vi "DSC Alarm Event Example.vi"() -> ()   [LabVIEW 2018, in "Dynamic Shared Variables.lvlib"]
uses:
  Dynamic Shared Variables.lvlib
  Alarm Cluster (UI).ctl
  Alarm Cluster.ctl
  <vilib>/Utility/miscctls.llb/LVMouseTypeDef.ctl
  Tag VIs/Tag FGV Operation Enum.ctl
  Alarm Log Operation Enum.ctl
  <vilib>/lvdsc/NI_DSC.lvlib
  Waveform Loop/Waveform Loop.lvlib
panel:
  out "Alarm CSV Logfile path":path
  out "Alarm Event Time":timestamp
  in  "Tag Value":dbl=80.0 format="%#_13g"
  in  "Write Tag Value":bool
  in  "numeric alarm settings":T1={"enable? (F)"=TRUE, "name"="HiHi", "alarm type"=enum."HI_HI", "level/change"=50.0, "deadband/time"=1.0, "priority"=1, "ack type"=enum."Each Occurrence", "area"="", "description"="", "log? (T)"=TRUE}
  in  "Create Shared Variable":bool
  out "Alarm Model":T2[](array[typedef]) {"Alarm"."value" format="%.2f"; "Alarm"."setpoint" format="%.2f"; "Alarm"."clear time" format="%<%X\n%x>T"; "Alarm"."ack time" format="%<%X\n%x>T"; "Alarm"."set time" format="%<%X\n%x>T"}
  in  "Alarms":T3[](array[typedef])
  in  "stop":bool
  # "Instructions\n1. Press Create Shared Variable button with designated HI_HI threshold.\n2. Press Write Tag Value to write a Tag Value that is above the HI_HI threshold.\n3. Observe that the Alarm Event was triggered when the Alarm Event Time changes.\n4. Observer that the HIHi alarm is displayed in the alarm array."
  # "2."
  # "1."
  # "3."
  # "4."
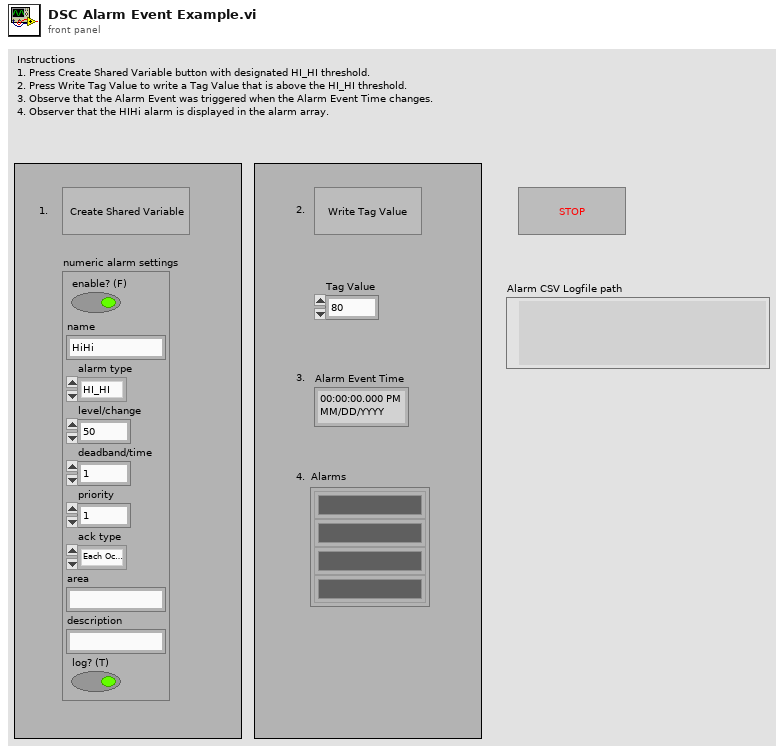
[diagram p1: front panel]
types:
  T1 = cluster{"enable? (F)":bool, "name":string, "alarm type":enum16{"HI_HI", "HI", "LO", "LO_LO"}, "level/change":dbl, "deadband/time":dbl, "priority":u32, "ack type":enum16{"Auto", "User", "None", "Each Occurrence"}, "area":string, "description":string, "log? (T)":bool}
  T2 = typedef "Dynamic Shared Variables.lvlib/Alarm Cluster.ctl" = cluster{"Color Box":u32, "Name":string, "Ack":bool, "Alarm":cluster{"alarm URL":string, "set time":timestamp, "set user":string, "ack time":timestamp, "ack user":string, "clear time":timestamp, "clear user":string, "setpoint":dbl, "value":dbl, "priority":u32, "alarm area":string, "alarm description":string, "ack comment":string, "event?":bool, "Refnum":u64}}
  T3 = typedef "Dynamic Shared Variables.lvlib/Alarm Cluster (UI).ctl" = cluster{"Color Box":u32, "Name":string, "Ack":bool}
  T4 = typedef "Alarm Log Operation Enum.ctl" = enum16{"Create Log", "Log Alarm", "Close Log"}
  T5 = typedef "Tag FGV Operation Enum.ctl" = enum16{"Init", "Set Notification Queue", "Create Tag", "Commit", "Write Tag (Numeric)", "Write Tag (Boolean)", "Read All Tags", "Read One Tag", "Delete Tag Category", "Set Alarm Parameters (Numeric)", "Set Alarm Parameters (Boolean)", "Enable All Alarms", "Disable All Alarms", "Delete All Tags", "Read Alarms", "Ack Alarm", "Read Alarm Parameters (Numeric)", "Read Alarm Parameters (Boolean)"}
  T6 = typedef "LVMouseTypeDef.ctl" = cluster{"Mouse Position":cluster{"X":i32, "Y":i32}, "Mouse Modifiers":cluster{"Button Down":bool, "Shift Mod":bool, "Menu Mod":bool, "Option Mod":bool}}
  T7 = cluster{"Down":bool, "Mouse":T6, "Drag":bool, "Canvas":bool}
  T8 = enum32{"u32BitField", "bool", "double", "string", "int8", "uint8", "int16", "uint16", "int32", "uint32", "int64", "uint64", "single", "double waveform", "int16 waveform", "array of boolean", "array of int8", "array of uint8", "array of int16", "array of uint16", "array of int32", "array of uint32", "array of int64", "array of uint64", "array of single", "array of double", "array of double waveform", "array of int16 waveform", "array of string", "variant", "timestamp", "fixed point", "custom"}
  T9 = cluster{"alarm URL":string, "set time":timestamp, "set user":string, "ack time":timestamp, "ack user":string, "clear time":timestamp, "clear user":string, "setpoint":dbl, "value":dbl, "priority":u32, "alarm area":string, "alarm description":string, "ack comment":string, "event?":bool, "Refnum":u64}[]
  T10 = cluster{"alarm URL":string, "set time":timestamp, "set user":string, "ack time":timestamp, "ack user":string, "clear time":timestamp, "clear user":string, "setpoint":dbl, "value":dbl, "priority":u32, "alarm area":string, "alarm description":string, "ack comment":string, "event?":bool, "Refnum":u64}
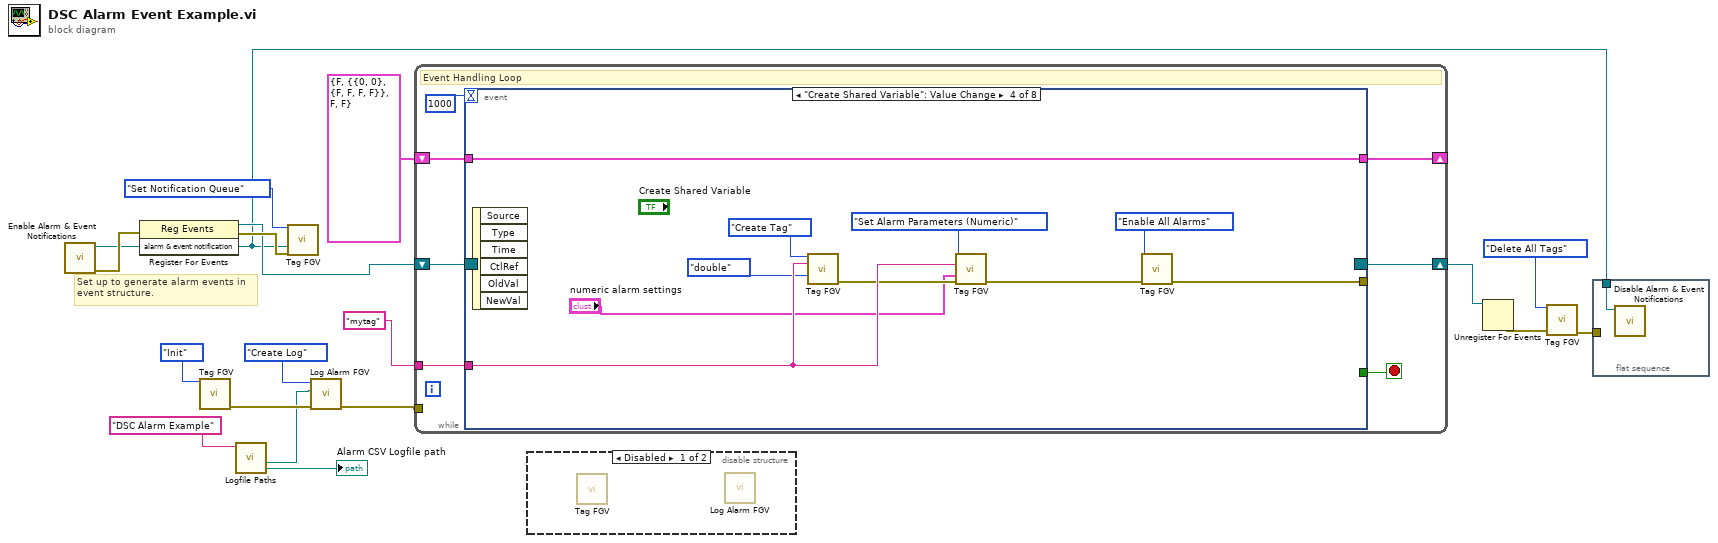
[diagram p0: block diagram]
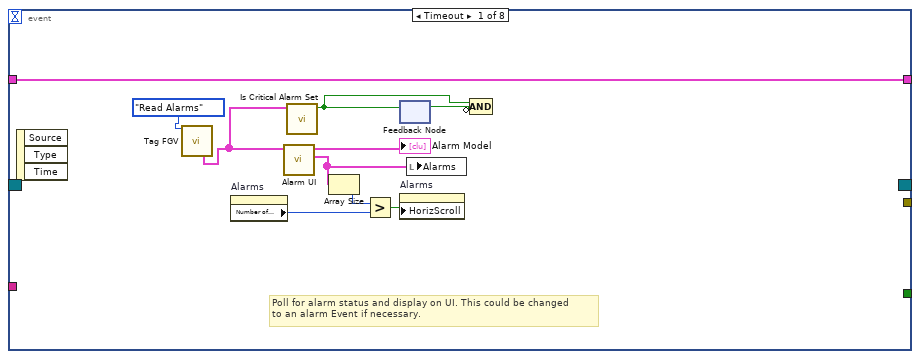
[diagram p3: hidden frame]
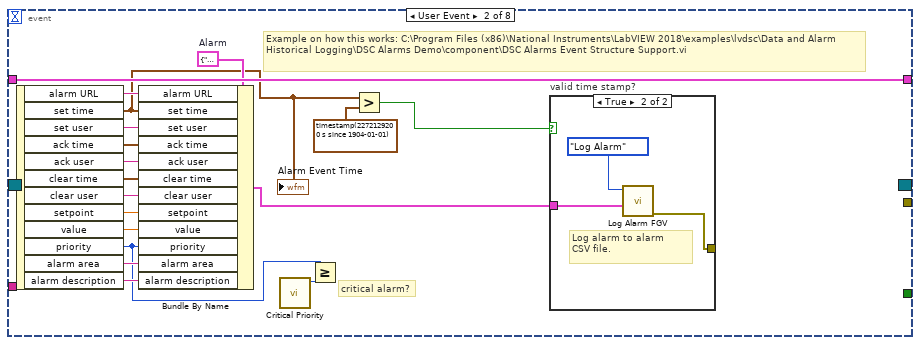
[diagram p4: hidden frame]
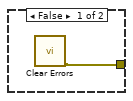
[diagram p5: hidden frame]
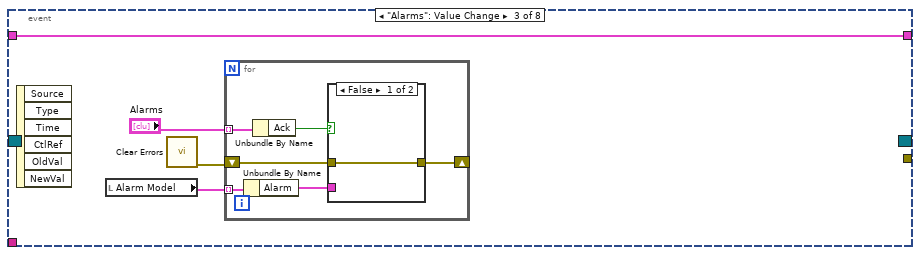
[diagram p6: hidden frame]
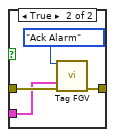
[diagram p7: hidden frame]
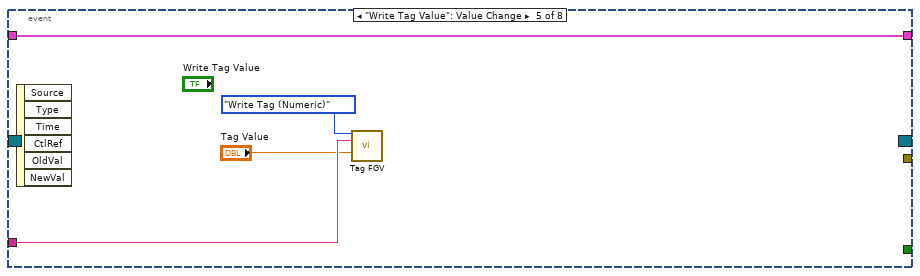
[diagram p8: hidden frame]
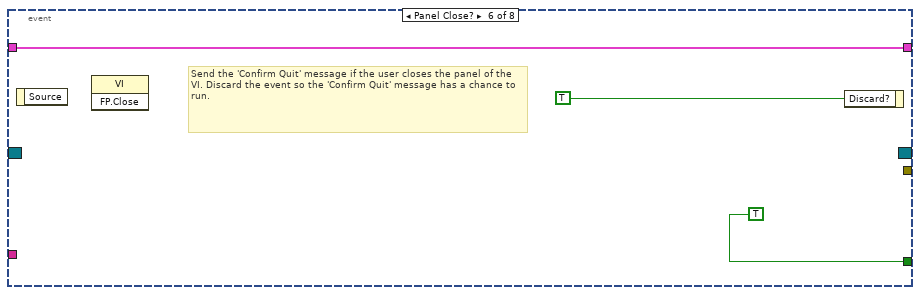
[diagram p9: hidden frame]
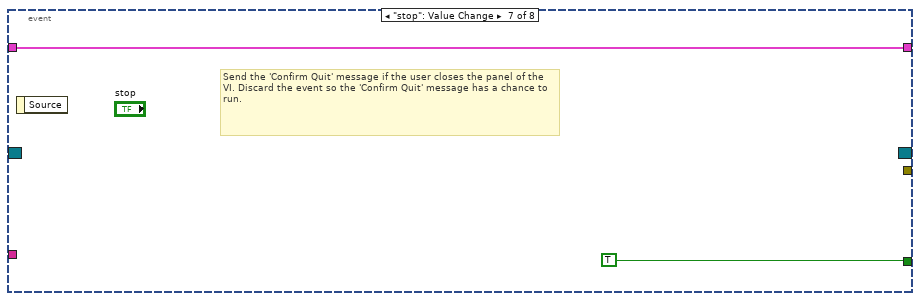
[diagram p10: hidden frame]
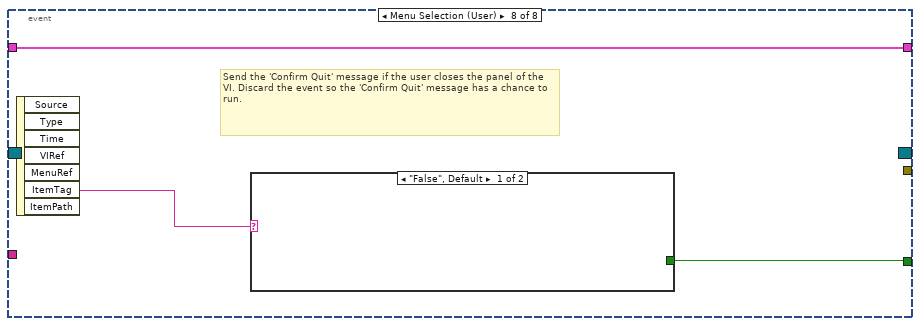
[diagram p11: hidden frame]
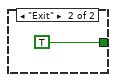
[diagram p12: hidden frame]
diagram:
  # "Set up to generate alarm events in\nevent structure."
  n1 = call <vilib>:"Enable Alarm & Event Notifications.vi"() -> ("error out"=w14:errorcluster, "alarm & event notification"=w2:refnum<user-event>)  [unwired: 10 in]
  n2 = register-events(error in=w14, w2) -> (reference out=w12:refnum<event-registration>, error out=w13:errorcluster)  [unwired: 1 in]
  n3 = call "Tag FGV.vi"("Operation"=Tag_FGV_Operation_Enum."Init") -> ("error out"=w6:errorcluster)  [unwired: 7 in, 7 out]
  n4 = call "Logfile Paths.vi"("File Name"="DSC Alarm Example") -> ("Alarm CSV Logfile path"=w3:path)  [unwired: 8 in, 2 out]
  "Alarm CSV Logfile path" <- w3
  n5 = call "Tag FGV.vi"("Operation"=Tag_FGV_Operation_Enum."Set Notification Queue", "Data"=w2, "error in (no error)"=w13) -> ()  [unwired: 5 in, 8 out]
  n6 = call "Log Alarm FGV.vi"("error in (no error)"=w6, "Path"=w3, "Operation"=Alarm_Log_Operation_Enum."Create Log") -> ("error out"=w5:errorcluster)  [unwired: 8 in]
  n7 = while {
    shift-right: [w22] -> w17
    shift-left: w12 -> [w24]
    shift-right: [w20] -> _
    shift-left: T7 {"Down"=FALSE, "Mouse"={"Mouse Position"={"X"=0, "Y"=0}, "Mouse Modifiers"={"Button Down"=FALSE, "Shift Mod"=FALSE, "Menu Mod"=FALSE, "Option Mod"=FALSE}}, "Drag"=FALSE, "Canvas"=FALSE} -> [w21]
    tunnel: "mytag" ("Tag Name") -> [w19]
    tunnel: w5 -> [_]
    stop <- w23 stop-if-true
    # "Event Handling Loop"
    n8 = event shown="[3] \"Create Shared Variable\": Value Change" {
      selector: w24 -> [_ _ _ _ _ _ _ _]
      dyn-events: [_ _ _ _ _ _ _ _] -> w22
      timeout: 1000 -> [_ _ _ _ _ _ _ _]
      tunnel: [_ _ _ _ _ TRUE TRUE w93] -> w23
      tunnel: w21 -> [w34 w52 w57 w81 w85 w86 w89 w92]
      tunnel: [w34 w52 w57 w81 w85 w86 w89 w92] -> w20
      tunnel: w19 -> [_ _ _ w78 w83 _ _ _]
      tunnel: [_ _ _ w72 _ _ _ _] -> _
      event Timeout {
        # "Poll for alarm status and display on UI. This could be changed\nto an alarm Event if necessary."
        n9 = event-data() -> ()  [unwired: 1 in, 3 out]
        n10 = call "Tag FGV.vi"("Operation"=Tag_FGV_Operation_Enum."Read Alarms") -> ("alarms"=w28:T9)  [unwired: 7 in, 7 out]
        n11 = property on="Alarms" class="Arr (strict)"() -> ("Number of Columns"=w31:u32)  [unwired: 2 in, 2 out]
        n12 = call "Alarm UI.vi"("alarms"=w28) -> ("UI Alarms"=w33:T3[], "Alarm Model"=→"Alarm Model":T2[])  [unwired: 9 in]
        n13 = call "Is Critical Alarm Set.vi"("alarms"=w28) -> ("critical alarm?"=w26:bool)  [unwired: 10 in]
        n14 = Array Size(array=w33) -> (size(s)=w32:i32)
        n15 = Greater?(x=w32, y=w31) -> (0:w30:bool)
        n16 = feedback #1() -> (w27:bool)  [unwired: 1 in]
        n17 = feedback-in #1(w26) -> ()
        n18 = property on="Alarms" class="Arr (strict)"("HorizScroll"=w30) -> ()  [unwired: 2 in, 2 out]
        n19 = local write "Alarms"(w33) -> ()
        n20 = Compound Arithmetic op=AND(w26, invert w27) -> ()  [unwired: 1 out]
      }
      event User Event {
        w50 = T10 {"alarm URL"="", "set time"=timestamp(0 s since 1904-01-01), "set user"="", "ack time"=timestamp(0 s since 1904-01-01), "ack user"="", "clear time"=timestamp(0 s since 1904-01-01), "clear user"="", "setpoint"=0.0, "value"=0.0, "priority"=0, "alarm area"="", "alarm description"="", "ack comment"="", "event?"=FALSE, "Refnum"=0}  # Alarm
        # "Example on how this works: C:\\Program Files (x86)\\National Instruments\\LabVIEW 2018\\examples\\lvdsc\\Data and Alarm Historical Logging\\DSC Alarms Demo\\component\\DSC Alarms Event Structure Support.vi"
        # "critical alarm?"
        n21 = event-data() -> ("alarm URL"=w49:string, "set time"=w48:timestamp, "set user"=w47:string, "ack time"=w46:timestamp, "ack user"=w45:string, "clear time"=w44:timestamp, "clear user"=w43:string, "setpoint"=w42:dbl, "value"=w41:dbl, "priority"=w38:u32, "alarm area"=w40:string, "alarm description"=w39:string)  [unwired: 1 in]
        "Alarm Event Time" <- w48
        n22 = Bundle By Name(cluster=w50, "alarm URL"=w49, "set time"=w48, "set user"=w47, "ack time"=w46, "ack user"=w45, "clear time"=w44, "clear user"=w43, "setpoint"=w42, "value"=w41, "priority"=w38, "alarm area"=w40, "alarm description"=w39) -> (w36:T10)
        n23 = call "Critical Priority.vi"() -> ("critical priority"=w37:i32)  [unwired: 11 in]
        n24 = Greater Or Equal?(x=w38, y=w37) -> ()  [unwired: 1 out]
        n25 = Greater?(x=w48, y=timestamp(2272129200 s since 1904-01-01)) -> (0:w35:bool)
        n26 = case "valid time stamp?" shown="True" w35 {
          tunnel: [w53 w54] -> _
          tunnel: w36 -> [_ w56]
          frame False {
            n27 = call <vilib>:"Clear Errors.vi"() -> ("error out"=w53:errorcluster)  [unwired: 6 in, 1 out]
          }
          frame True {
            # "Log alarm to alarm\nCSV file."
            n28 = call "Log Alarm FGV.vi"("Alarm"=w56, "Operation"=Alarm_Log_Operation_Enum."Log Alarm") -> ("error out"=w54:errorcluster)  [unwired: 9 in]
          }
        }
      }
      event "Alarms": Value Change {
        n29 = event-data() -> ()  [unwired: 1 in, 6 out]
        n30 = local read "Alarm Model"() -> (w59:T2[])
        n31 = call <vilib>:"Clear Errors.vi"() -> ("error out"=w58:errorcluster)  [unwired: 6 in, 1 out]
        n32 = for {
          shift-right: [w65] -> _
          shift-left: w58 -> [w66]
          tunnel: "Alarms" -> [w64] mode=indexing
          tunnel: w59 -> [w62] mode=indexing
          n33 = Unbundle By Name(w62) -> ("Alarm"=w61:T10)
          n34 = Unbundle By Name(w64) -> ("Ack"=w63:bool)
          n35 = case shown="False" w63 {
            tunnel: w66 -> [w67 w71]
            tunnel: [w67 w70] -> w65
            tunnel: w61 -> [_ w68]
            frame False {
            }
            frame True {
              n36 = call "Tag FGV.vi"("Operation"=Tag_FGV_Operation_Enum."Ack Alarm", "Data"=w68, "error in (no error)"=w71) -> ("error out"=w70:errorcluster)  [unwired: 5 in, 7 out]
            }
          }
        }
      }
      event "Create Shared Variable": Value Change {
        n37 = event-data() -> ()  [unwired: 1 in, 6 out]
        n38 = call "Tag FGV.vi"("Operation"=Tag_FGV_Operation_Enum."Create Tag", "Tag Name"=w78, "Data"=T8."double" ("data type")) -> ("error out"=w77:errorcluster)  [unwired: 5 in, 7 out]
        n39 = call "Tag FGV.vi"("Operation"=Tag_FGV_Operation_Enum."Set Alarm Parameters (Numeric)", "Tag Name"=w78, "Data"="numeric alarm settings", "error in (no error)"=w77) -> ("error out"=w74:errorcluster)  [unwired: 4 in, 7 out]
        n40 = call "Tag FGV.vi"("Operation"=Tag_FGV_Operation_Enum."Enable All Alarms", "error in (no error)"=w74) -> ("error out"=w72:errorcluster)  [unwired: 6 in, 7 out]
      }
      event "Write Tag Value": Value Change {
        n41 = event-data() -> ()  [unwired: 1 in, 6 out]
        n42 = call "Tag FGV.vi"("Operation"=Tag_FGV_Operation_Enum."Write Tag (Numeric)", "Tag Name"=w83, "Data"="Tag Value") -> ()  [unwired: 5 in, 8 out]
      }
      event Panel Close? {
        # "Send the 'Confirm Quit' message if the user closes the panel of the VI. Discard the event so the 'Confirm Quit' message has a chance to run."
        n43 = event-data() -> ()  [unwired: 1 in, 1 out]
        n44 = invoke class="VI" method="FP.Close"() -> ()  [unwired: 3 in, 3 out]
        n45 = event-data("Discard?"=TRUE) -> ()  [unwired: 1 in, 1 out]
      }
      event "stop": Value Change {
        # "Send the 'Confirm Quit' message if the user closes the panel of the VI. Discard the event so the 'Confirm Quit' message has a chance to run."
        n46 = event-data() -> ()  [unwired: 1 in, 1 out]
      }
      event Menu Selection (User) {
        # "Send the 'Confirm Quit' message if the user closes the panel of the VI. Discard the event so the 'Confirm Quit' message has a chance to run."
        n47 = event-data() -> ("ItemTag"=w91:string)  [unwired: 1 in, 6 out]
        n48 = case shown="\"False\", Default" w91 {
          tunnel: [_ TRUE] -> w93
          frame "False", Default {
          }
          frame "Exit" {
          }
        }
      }
    }
  }
  n49 = disable-structure shown="Disabled" {
    frame Disabled {
      n50 = call "Tag FGV.vi"() -> ()  [unwired: 8 in, 8 out]
      n51 = call "Log Alarm FGV.vi"() -> ()  [unwired: 11 in, 1 out]
    }
    frame Enabled {
    }
  }
  n52 = Unregister For Events(event registration refnum=w17) -> (error out=w8:errorcluster)  [unwired: 1 in]
  n53 = call "Tag FGV.vi"("Operation"=Tag_FGV_Operation_Enum."Delete All Tags", "error in (no error)"=w8) -> ("error out"=w1:errorcluster)  [unwired: 6 in, 7 out]
  n54 = flat-sequence {
    tunnel: w2 -> [w95]
    tunnel: w1 -> [_]
    frame #0 {
      n55 = call <vilib>:"Disable Alarm & Event Notifications.vi"("notification refnum"=w95) -> ()  [unwired: 10 in, 1 out]
    }
  }
